vi "Analyze & Present Data.vi"(1 "데이터":waveform(dbl)(graph)={"t0"=timestamp(22.93120638085739 s since 1904-01-01), "dt"=0.0009970089730807576, "Y"=array[500 elements]}) -> ()   [LabVIEW 2010]
doc: "이 VI는 LabVIEW Core II 교육과정의 연습문제 4-3에 대한 솔루션입니다.\n\n이 VI는 웨이브폼 그래프 커서 속성을 사용하여 그래프에서 볼 수 있는 데이터의 서브셋을 선택하고 이 데이터를 분석할 수 있습니다. 로그 결과를 파일로 버튼을 눌러서 분석 결과를 파일에 저장할 수 있습니다."
uses:
  <vilib>/measure/matone.llb/Extract Single Tone Information 1 Chan.vi
  <vilib>/measure/madcrms.llb/Basic Averaged DC-RMS for 1 Chan.vi
  <vilib>/measure/NI_MAPro.lvlib
panel:
  out "분석 결과":T1 {"Phase (deg)" format="%0.2f"; "Amplitude" format="%0.2f"; "DC Value" format="%0.2f"; "Frequency" format="%0.2f"; "RMS Value" format="%0.2f"}
  in  "초기 클러스터":T1={"Waveform Subset"={"t0"=timestamp(0 s since 1904-01-01), "dt"=0.0, "Y"=[]}, "DC Value"=0.0, "RMS Value"=0.0, "Frequency"=0.0, "Amplitude"=0.0, "Phase (deg)"=0.0, "No. of Points in Subset"=0} {"Phase (deg)" format="%0.2f"; "Amplitude" format="%0.2f"; "DC Value" format="%0.2f"; "Frequency" format="%0.2f"; "RMS Value" format="%0.2f"}
  in  "클러스터":cluster{"Analyze Data":bool, "Return":bool}
  # "그래프에서 노란색 세로 선 사이의 부분이 분석됩니다.  이 노란색 세로 선을 끌어 분석되는 부분을 변경할 수 있습니다.  데이터를 분석하고 분석 결과 아래에 결과를 나타내려면 선택 부분 분석 버튼을 누릅니다.  완료시 리턴 버튼을 누릅니다."
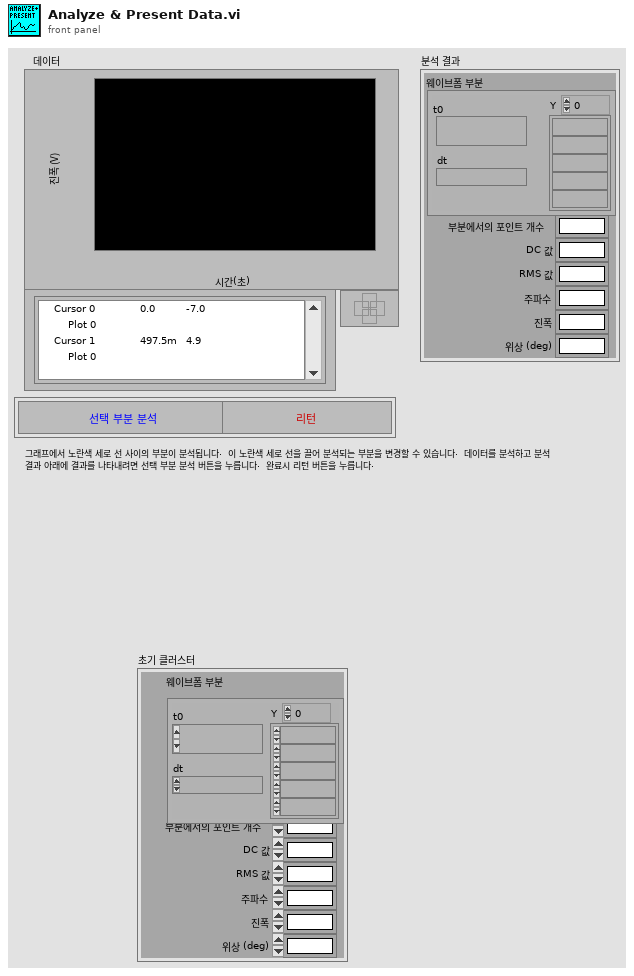
[diagram p1: front panel]
types:
  T1 = cluster{"Waveform Subset":waveform(dbl), "DC Value":dbl, "RMS Value":dbl, "Frequency":dbl, "Amplitude":dbl, "Phase (deg)":dbl, "No. of Points in Subset":i32}
  T2 = cluster{"데이터":waveform(dbl), "DC value":dbl, "RMS value":dbl, "detected frequency":dbl, "detected amplitude":dbl, "detected phase (deg)":dbl, i32}
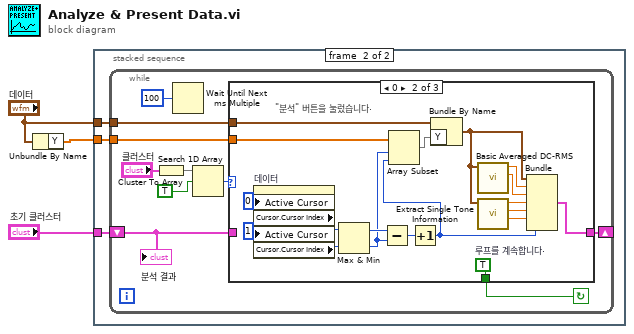
[diagram p0: block diagram]
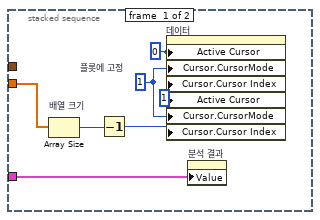
[diagram p2: hidden frame]
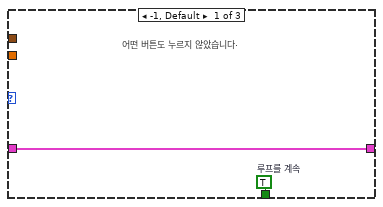
[diagram p3: hidden frame]
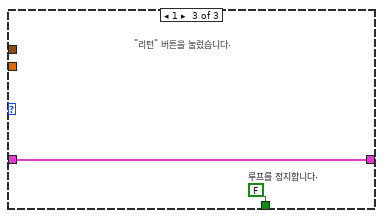
[diagram p4: hidden frame]
diagram:
  n1 = Unbundle By Name("데이터") -> ("Y"=w1:dbl[])
  n2 = stacked-sequence {
    tunnel: "데이터" -> [_ w13]
    tunnel: "초기 클러스터" -> [w5 w12]
    tunnel: w1 -> [w9 w11]
    frame #0 {
      w7 = u32 1  # 플롯에 고정
      w4 = u32 0 ("Active Cursor")
      n3 = Array Size "배열 크기"(array=w9) -> (size(s)=w10:i32)
      n4 = Decrement(x=w10) -> (x-1=w6:i32)
      n5 = property on="데이터" class="WFGraph (엄격한)"("Active Cursor"=w4, "Cursor.CursorMode"=w7, "Cursor.Cursor Index"=w4, "Active Cursor"=u32 1, "Cursor.CursorMode"=w7, "Cursor.Cursor Index"=w6) -> ()  [unwired: 2 in, 2 out]
      n6 = property on="분석 결과" class="Clust (엄격한)"("Value"=w5) -> ()  [unwired: 2 in, 2 out]
    }
    frame #1 {
      n7 = while {
        tunnel: w11 -> [w15]
        tunnel: w13 -> [w16]
        shift-left: w12 -> [w17]
        shift-right: [w21] -> _
        stop <- w20 continue-if-true
        n8 = Cluster To Array(cluster="클러스터") -> (array=w23:bool[])
        n9 = Wait Until Next ms Multiple(millisecond multiple=u32 100) -> ()  [unwired: 1 out]
        n10 = Search 1D Array ("Search\n1D Array")(1D array=w23, element=TRUE) -> (index of element=w19:i32)  [unwired: 1 in]
        n11 = case shown="0" w19 {
          tunnel: [w25 w41 w46] -> w21
          tunnel: w17 -> [w25 _ w46]
          tunnel: [w24 w42 w45] -> w20
          tunnel: w16 -> [_ w34 _]
          tunnel: w15 -> [_ w28 _]
          frame -1, Default {
            w24 = TRUE  # 루프를 계속
            # "어떤 버튼도 누르지 않았습니다."
          }
          frame 0 {
            w42 = TRUE  # 루프를 계속합니다.
            # "\"분석\" 버튼을 눌렀습니다."
            n12 = property on="데이터" class="WFGraph (엄격한)"("Active Cursor"=u32 0, "Active Cursor"=u32 1) -> ("Cursor.Cursor Index"=w30:i32, "Cursor.Cursor Index"=w29:i32)  [unwired: 2 in, 2 out]
            n13 = Max & Min(x=w30, y=w29) -> (max(x,y)=w44:i32, min(x,y)=w43:i32)
            n14 = Subtract(x=w44, y=w43) -> (x-y=w33:i32)
            n15 = Increment(x=w33) -> (x+1=w26:i32)
            n16 = Array Subset(array=w28, index=w43, length=w26) -> (w35:dbl[])
            n17 = Bundle By Name(cluster=w34, "Y"=w35) -> (w27:waveform(dbl))
            n18 = call-poly <vilib>:"Basic Averaged DC-RMS.vi"("signal in"=w27) -> ("RMS value"=w39:dbl, "DC value"=w40:dbl)  [unwired: 7 in, 2 out]
            n19 = call-poly <vilib>:"Extract Single Tone Information.vi"("time signal in"=w27) -> ("detected phase (deg)"=w36:dbl, "detected amplitude"=w37:dbl, "detected frequency"=w38:dbl)  [unwired: 5 in, 3 out]
            n20 = Bundle "Bundle"("데이터"=w27, "DC value"=w40, "RMS value"=w39, "detected frequency"=w38, "detected amplitude"=w37, "detected phase (deg)"=w36, w26) -> (w41:T2)  [unwired: 1 in]
          }
          frame 1 {
            w45 = FALSE  # 루프를 정지합니다.
            # "\"리턴\" 버튼을 눌렀습니다."
          }
        }
        "분석 결과" <- w17
      }
    }
  }
